vi "Read channel.vi"(8 "error in (no error)":errorcluster caption="에러 입력(에러 없음)", 11 "Waveform File 입력":refnum<class "Waveform File.lvclass">) -> (0 "error out":errorcluster caption="에러 출력", 2 "channel":i32, 3 "Waveform File 출력":refnum<class "Waveform File.lvclass">)   [LabVIEW 2020, in "Waveform File.lvclass"]
uses:
  Waveform File.lvclass
  Waveform File.lvclass/Waveform File.ctl
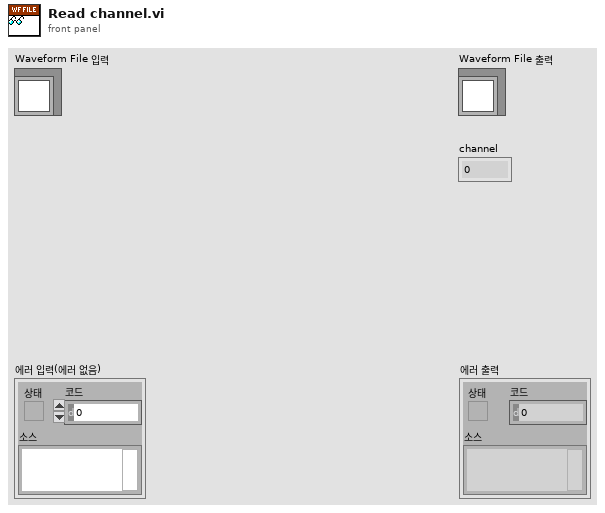
[diagram p1: front panel]
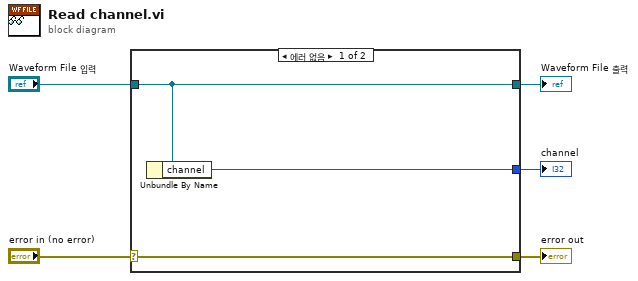
[diagram p0: block diagram]
diagram:
  n1 = case shown="에러 없음" "error in (no error)" {
    selector: "error in (no error)" -> [w8 w9]
    tunnel: [w8 w9] -> w4
    tunnel: [w7 w10] -> w2
    tunnel: "Waveform File 입력" -> [w7 w10]
    tunnel: [w6 _] -> w1
    frame No Error {
      n2 = Unbundle By Name(w7) -> ("channel"=w6:i32)
    }
    frame Error {
    }
  }
  "error out" <- w4
  "Waveform File 출력" <- w2
  "channel" <- w1
